vi "Result_CSVSave.vi"(11 "YTESTER测试数据":T1 caption="不要修改！") -> (3 "YTESTER结论":T2)   [LabVIEW 2017]
doc: "VIDescription=CSV格式的本地保存。"
uses:
  YtCommon.lvlibp/yt`Step StepBaseInput.ctl
  YtCommon.lvlibp/yt`Step StepResult.ctl
  YtCommon.lvlibp/yt`Step TestData.ctl
  YtCommon.lvlibp/yt`Step System Queue.ctl
  ccbe6eb8-0466-4861-8968-f05c08307fff.vi
  ac0dbf41-8066-48af-8511-23b2e407a70c.vi
  b6c5d7ee-a3f7-45be-aa43-2dbab6f386c4.vi
  YtCommon.lvlibp/yt`varSystemlib IO Read Variable.vi
  YtCommon.lvlibp
  kernel32.dll
  Advapi32.dll
panel:
  out "TiTles Array":string[](array[string])
  out "DATA array":string[](array[string])
  in  "debug":bool
  out "debug TestTable":string[][](table)
  in  "YTESTER开放参数":cluster{"YTESTER_BaseInput":T3, "保存路径":path}={"YTESTER_BaseInput"={"isTest"=FALSE, "isSkip"=FALSE, "StepName"="CSV式保存", "OnPass"=enum."Next", "OnFail"=enum."Next", "ReTestNumber"=0.0}, "保存路径"=path ""}
  # "CSV格式保存（本地）"
  # "改重入VI了！每个Socket写不同文件！"
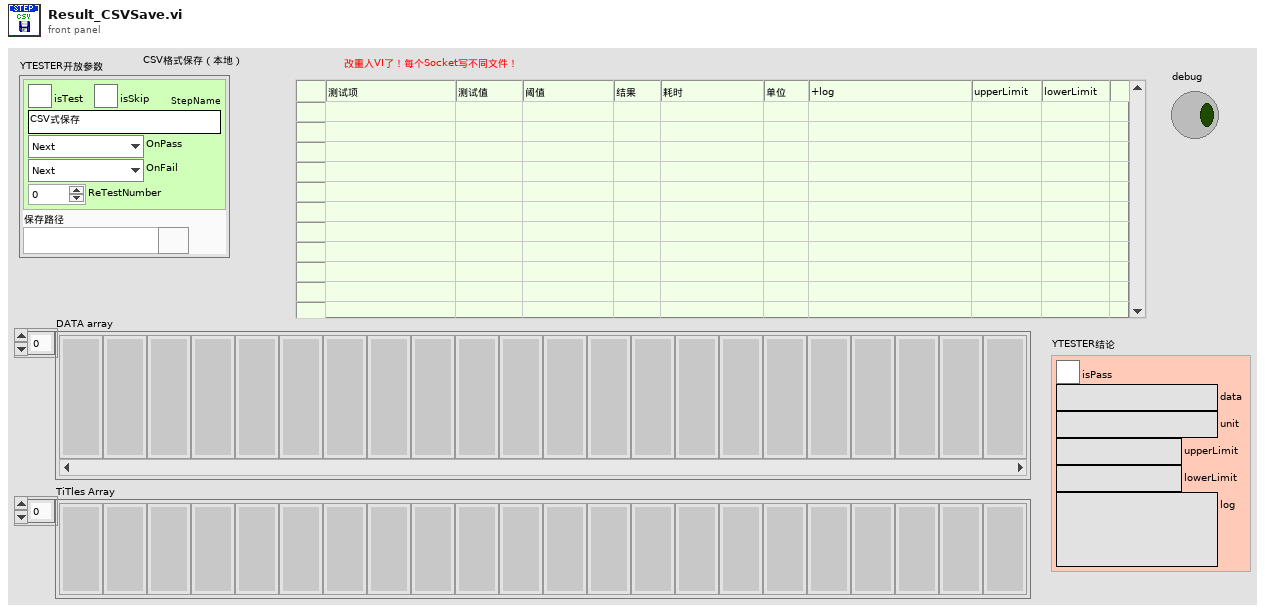
[diagram p1: front panel]
types:
  T1 = typedef "YtCommon.lvlibp/yt`Step TestData.ctl" = cluster{"Socket(From1)":i32, "SN":refnum<notifier>, "StopFlagRef":refnum<notifier>, "YT System Queue":refnum<queue>}
  T2 = typedef "YtCommon.lvlibp/yt`Step StepResult.ctl" = cluster{"isPass":bool, "data":string, "unit":string, "upperLimit":string, "lowerLimit":string, "log":string}
  T3 = typedef "YtCommon.lvlibp/yt`Step StepBaseInput.ctl" = cluster{"isTest":bool, "isSkip":bool, "StepName":string, "OnPass":enum16{"Next", "ToOVER", "Terminate"}, "OnFail":enum16{"Next", "ToOVER", "Terminate"}, "ReTestNumber":dbl}
  T4 = enum16{"open", "replace", "create", "open or create", "replace or create", "replace or create with confirmation"}
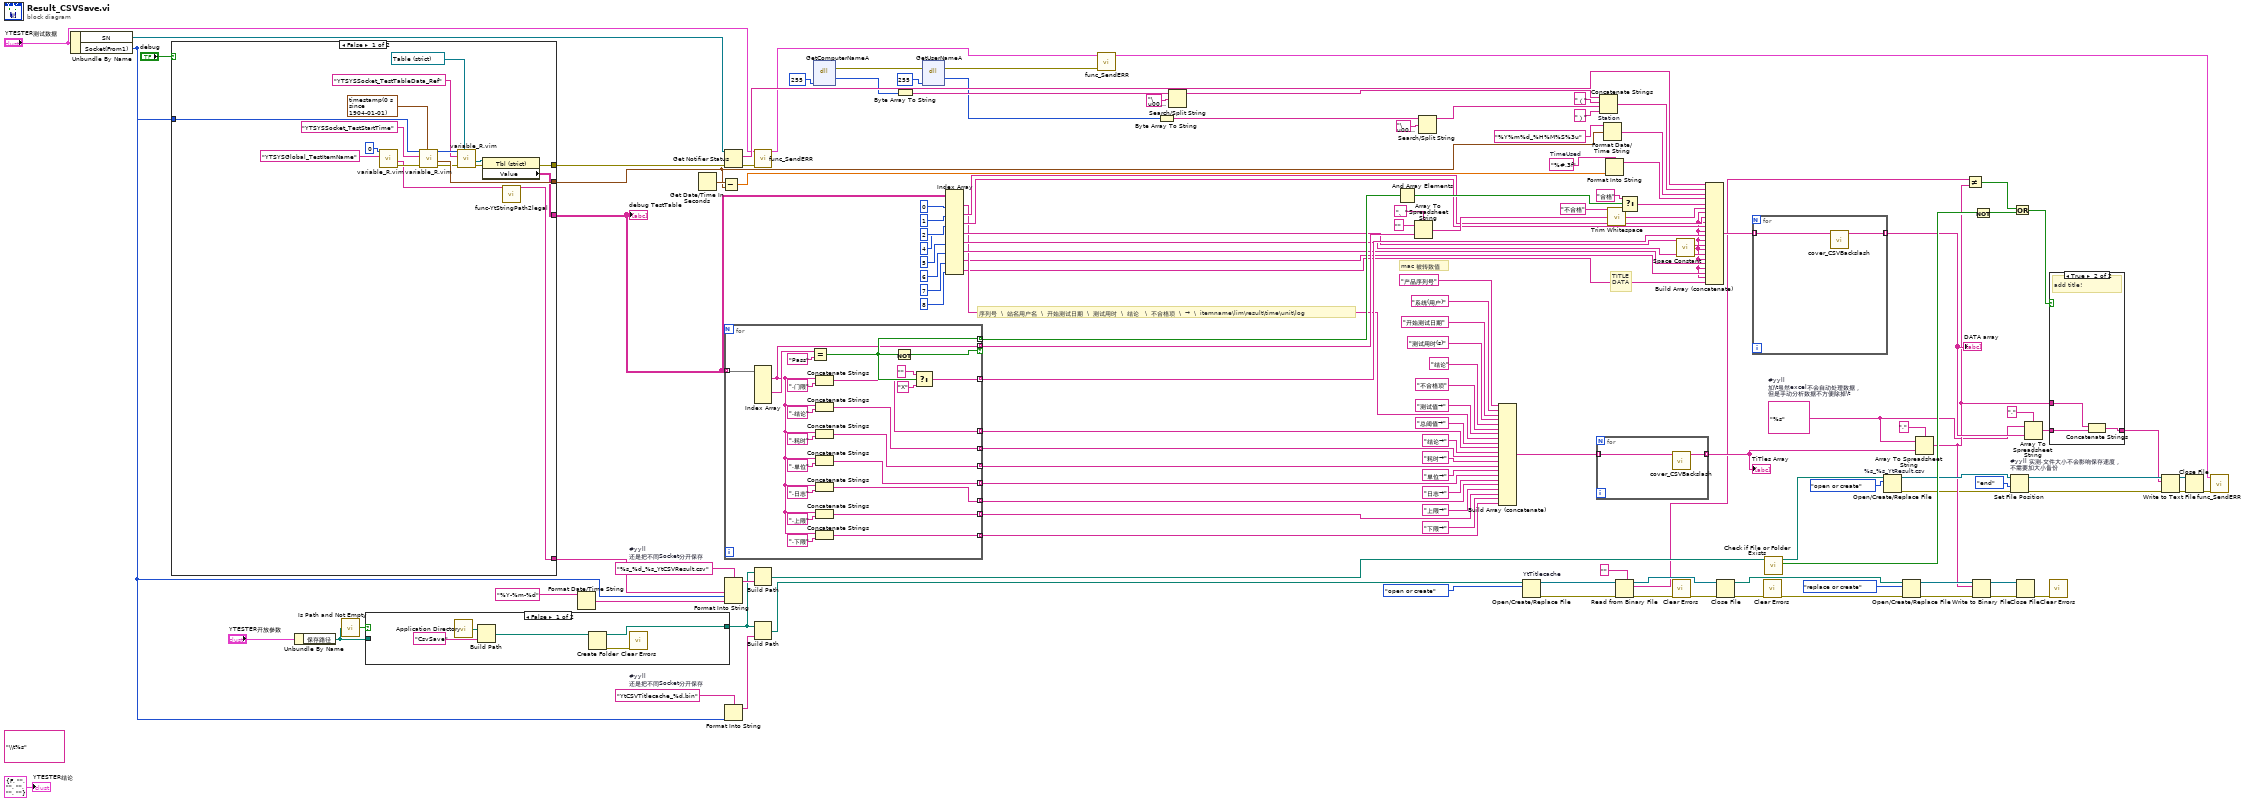
[diagram p0: block diagram]
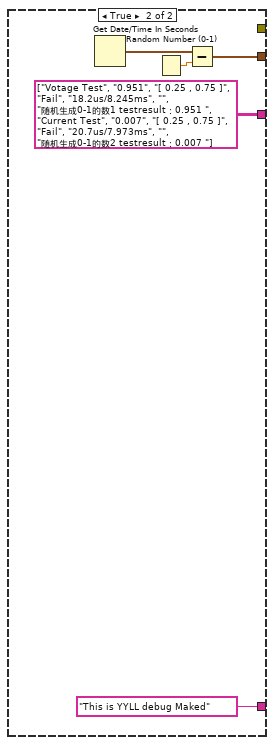
[diagram p2: hidden frame]
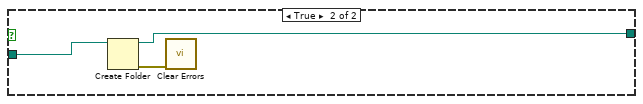
[diagram p4: hidden frame]
diagram:
  (unwired) "\\t%s" ("format string")
  w3 = "YtCSVTitlecache_%d.bin"  # #yyll 还是把不同Socket分开保存
  w15 = "%s"  # #yyll  加\t虽然excel不会自动处理数据， 但是手动分析数据不方便除掉\t
  w74 = "%s_%d_%s_YtCSVResult.csv"  # #yyll 还是把不同Socket分开保存
  w103 = "%#.3f"  # TimeUsed
  # "mac 被转数值"
  # "序列号  \\  站名用户名  \\  开始测试日期  \\  测试用时  \\  结论   \\  不合格项  \\  →  \\  itemname\\lim\\result\\time\\unit\\log"
  # "TITLE\nDATA"
  n1 = Unbundle By Name("YTESTER测试数据") -> ("SN"=w22:refnum<notifier>, "Socket(From1)"=w1:i32)
  n2 = case shown="False" "debug" {
    tunnel: [w153 "This is YYLL debug Maked"] -> w72
    tunnel: w1 -> [w152 _]
    tunnel: [w149 w156] -> w26
    tunnel: [w143 string[][] [["Votage Test", "0.951", "[ 0.25 , 0.75 ]", "Fail", "18.2us/8.245ms", "", "随机生成0-1的数1 testresult：0.951 "], ["Current Test", "0.007", "[ 0.25 , 0.75 ]", "Fail", "20.7us/7.973ms", "", "随机生成0-1的数2 testresult：0.007 "]] ("debug TestTable 2")] -> w25
    tunnel: [w137 _] -> w23
    frame False {
      n3 = call "variable_R.vim"("待获取变量名称"="YTSYSGlobal_TestItemName", "函数池名称"=0) -> ("error out"=w140:errorcluster, "value"=w138:string)  [unwired: 5 in, 3 out]
      n4 = call "variable_R.vim"("type"=timestamp(0 s since 1904-01-01), "error in"=w140, "待获取变量名称"="YTSYSSocket_TestStartTime", "函数池名称"=w152) -> ("error out"=w139:errorcluster, "value"=w149:timestamp, "函数池名称out"=w148:i32)  [unwired: 3 in, 2 out]
      n5 = call "variable_R.vim"("type"=refnum<vi> refnum ("TestTable"), "error in"=w139, "待获取变量名称"="YTSYSSocket_TestTableData_Ref", "函数池名称"=w148) -> ("error out"=w144:errorcluster, "value"=w145:refnum<vi>)  [unwired: 3 in, 3 out]
      n6 = property class="Tbl (strict)"(reference=w145, error in=w144) -> (error out=w137:errorcluster, "Value"=w143:string[][])  [unwired: 1 out]
      n7 = call "func-YtStringPath2legal.vi"("StringPath in"=w138) -> ("StringPath out"=w153:string)  [unwired: 10 in]
    }
    frame True {
      n8 = Get Date/Time In Seconds() -> (seconds since 1Jan1904=w158:timestamp)
      n9 = Random Number (0-1)() -> (number: 0 to 1=w157:dbl)
      n10 = Subtract(x=w158, y=w157) -> (x-y=w156:timestamp)
    }
  }
  "debug TestTable" <- w25
  n11 = Unbundle By Name("YTESTER开放参数") -> ("保存路径"=w133:path)
  n12 = call <vilib>:"Is Path and Not Empty.vi"("path"=w133) -> ("Is Path and Not Empty?"=w134:bool)  [unwired: 4 in]
  n13 = case shown="False" w134 {
    tunnel: w133 -> [_ w166]
    tunnel: [w160 w164] -> w38
    frame False {
      n14 = call <vilib>:"Application Directory.vi"() -> ("Application Directory"=w161:path)
      n15 = Build Path(base path=w161, name or relative path="CsvSave") -> (appended path=w163:path)
      n16 = Create Folder(path (use dialog)=w163) -> (created path=w160:path, error out=w159:errorcluster)  [unwired: 2 in, 1 out]
      n17 = call <vilib>:"Clear Errors.vi"("error in (no error)"=w159) -> ()  [unwired: 5 in, 2 out]
    }
    frame True {
      n18 = Create Folder(path (use dialog)=w166) -> (created path=w164:path, error out=w165:errorcluster)  [unwired: 2 in, 1 out]
      n19 = call <vilib>:"Clear Errors.vi"("error in (no error)"=w165) -> ()  [unwired: 5 in, 2 out]
    }
  }
  n20 = Format Date/Time String(time format string (%c)="%Y-%m-%d") -> (date/time string=w4:string)  [unwired: 1 in, 1 out]
  n21 = Get Date/Time In Seconds() -> (seconds since 1Jan1904=w105:timestamp)
  n22 = Subtract(x=w105, y=w26) -> (x-y=w104:dbl)
  n23 = Get Notifier Status(notifier=w22, error in (no error)=w23) -> (current notification=w127:string, error out=w128:errorcluster)  [unwired: 3 out]
  n24 = for {
    tunnel: w25 -> [w189] mode=indexing
    tunnel: [w185] -> w129 mode=indexing
    tunnel: [w169] -> w125 mode=indexing if=w186
    tunnel: [w182] -> w96 mode=indexing
    tunnel: [w176] -> w79 mode=indexing
    tunnel: [w175] -> w78 mode=indexing
    tunnel: [w174] -> w77 mode=indexing
    tunnel: [w173] -> w76 mode=indexing
    tunnel: [w172] -> w75 mode=indexing
    tunnel: [w168] -> w21 mode=indexing
    tunnel: [w167] -> w20 mode=indexing
    n25 = Index Array(array=w189) -> (element #1=w169:string, element #4=w188:string)  [unwired: 6 in, 4 out]
    n26 = Equal?(x=w188, y="Pass") -> (x = y?=w185:bool)
    n27 = Concatenate Strings(w169, ".门限" ("string")) -> (w176:string)
    n28 = Concatenate Strings(w169, ".结论" ("string")) -> (w175:string)
    n29 = Concatenate Strings(w169, ".耗时" ("string")) -> (w174:string)
    n30 = Concatenate Strings(w169, ".单位" ("string")) -> (w173:string)
    n31 = Concatenate Strings(w169, ".日志" ("string")) -> (w172:string)
    n32 = Concatenate Strings(w169, ".上限" ("string")) -> (w168:string)
    n33 = Concatenate Strings(w169, ".下限" ("string")) -> (w167:string)
    n34 = Not(x=w185) -> (.not. x?=w186:bool)
    n35 = Select(t="" ("y"), s=w185, f="Ⅹ" ("y")) -> (s? t:f=w182:string)
  }
  n36 = Format Into String(format string=w74, w72, w1, w4) -> (resulting string=w71:string)  [unwired: 2 in, 1 out]
  n37 = Format Into String(format string=w3, w1) -> (resulting string=w2:string)  [unwired: 2 in, 1 out]
  n38 = call "func_SendERR.vi"("ERR (String\\Errclust)"=w128, "YTESTER测试数据 in"="YTESTER测试数据") -> ("YTESTER测试数据 out"=w31:T1)  [unwired: 9 in]
  n39 = Build Path(base path=w38, name or relative path=w71) -> (appended path=w60:path)
  n40 = Build Path(base path=w38, name or relative path=w2) -> (appended path=w39:path)
  n41 = dll-call lib="kernel32.dll" fn="GetComputerNameA" label="Get Computer Name"("size"=255) -> (error out=w33:errorcluster, "lpBuffer"=w120:u8[])  [unwired: 6 in, 1 out]
  n42 = Byte Array To String(unsigned byte array=w120) -> (string=w119:string)
  n43 = dll-call lib="advapi32.dll" fn="GetUserNameA" label="GetUserName"(error in=w33, "nSize"=u32 255) -> (error out=w32:errorcluster, "lpBuffer"=w116:u8[])  [unwired: 5 in, 1 out]
  n44 = Index Array(array=w25, index (col) #1=0 ("disabled index (col)"), index (col) #2=1 ("index (col)"), index (col) #3=2 ("index (col)"), index (col) #4=4 ("index (col)"), index (col) #5=5 ("index (col)"), index (col) #6=6 ("index (col)"), index (col) #7=7 ("index (col)"), index (col) #8=8 ("index (col)")) -> (element #1=w80:string[], element #2=w99:string[], element #3=w97:string[], element #4=w94:string[], element #5=w91:string[], element #6=w90:string[], element #7=w17:string[], element #8=w16:string[])  [unwired: 8 in]
  n45 = call "func_SendERR.vi"("ERR (String\\Errclust)"=w32, "YTESTER测试数据 in"=w31) -> ("YTESTER测试数据 out"=w30:T1)  [unwired: 9 in]
  n46 = Byte Array To String(unsigned byte array=w116) -> (string=w115:string)
  n47 = Search/Split String(string=w119, search string/char (-)="\u0000" ("regular expression")) -> (substring before match=w112:string)  [unwired: 1 in, 2 out]
  n48 = And Array Elements(Boolean array=w129) -> (logical AND=w132:bool)
  n49 = Array To Spreadsheet String(delimiter (Tab)="、", array=w125, 3:"" ("format string")) -> (spreadsheet string=w122:string)
  n50 = Search/Split String(string=w115, search string/char (-)="\u0000" ("regular expression")) -> (substring before match=w110:string)  [unwired: 1 in, 2 out]
  n51 = Build Array (concatenate) ("Build DATA Array")("产品序列号", "系统(用户)", "开始测试日期", "测试用时(s)", "结论", "不合格项", "测试值→", w80, "总阈值→", w79, "结论→", w78, "耗时→", w77, "单位→", w76, "日志→", w75, "上限→", w21, "下限→", w20) -> (w87:string[])
  n52 = Open/Create/Replace File "YtTitlecache"(file path (use dialog)=w39, operation (0:open)=T4."open or create") -> (refnum out=w51:refnum<file>, error out=w54:errorcluster)  [unwired: 4 in, 1 out]
  n53 = for {
    tunnel: [w191] -> w55 mode=indexing
    tunnel: w87 -> [w190] mode=indexing
    n54 = call "cover_CSVBackslash.vi"("String in"=w190) -> ("String out"=w191:string)  [unwired: 10 in]
  }
  "TiTles Array" <- w55
  n55 = Concatenate Strings "Station"(w112, "（" ("string"), w110, "）" ("string")) -> (w108:string)
  n56 = Format Date/Time String(time format string (%c)="%Y%m%d_%H%M%S%3u", seconds (now)=w26) -> (date/time string=w106:string)  [unwired: 1 in]
  n57 = Format Into String(format string=w103, w104) -> (resulting string=w102:string)  [unwired: 2 in, 1 out]
  n58 = call <vilib>:"Trim Whitespace.vi"("string"=w122) -> ("trimmed string"=w121:string)  [unwired: 1 in]
  n59 = Read from Binary File(5:"", 8:w54, 11:w51) -> (0:w48:errorcluster, 2:w36:string, 3:w49:refnum<file>)  [unwired: 3 in, 1 out]
  n60 = Select(t="合格", s=w132, f="不合格") -> (s? t:f=w126:string)
  n61 = call <vilib>:"Clear Errors.vi"("error in (no error)"=w48) -> ("error out"=w43:errorcluster)  [unwired: 5 in, 1 out]
  n62 = call <vilib>:"Space Constant.vi"() -> ("String"=w7:string)
  n63 = Build Array (concatenate) ("Build DATA Array")(w127, w108, w106, w102, w126, w121, w7, w99, w7, w97, w7, w96, w7, w94, w7, w91, w7, w90, w7, w17, w7, w16) -> (w89:string[])
  n64 = Close File(refnum=w49, error in=w43) -> (path=w46:path, error out=w41:errorcluster)
  n65 = for {
    tunnel: w89 -> [w193] mode=indexing
    tunnel: [w192] -> w58 mode=indexing
    n66 = call "cover_CSVBackslash.vi"("String in"=w193) -> ("String out"=w192:string)  [unwired: 10 in]
  }
  "DATA array" <- w58
  n67 = call <vilib>:"Clear Errors.vi"("error in (no error)"=w41) -> ("error out"=w40:errorcluster)  [unwired: 5 in, 1 out]
  n68 = call <vilib>:"Check if File or Folder Exists.vi"("path"=w60) -> ("file or folder exists?"=w67:bool, "dup path"=w66:path)  [unwired: 8 in, 1 out]
  n69 = Open/Create/Replace File "%s_%s_YtResult.csv"(file path (use dialog)=w66, operation (0:open)=T4."open or create") -> (refnum out=w65:refnum<file>, error out=w29:errorcluster)  [unwired: 4 in, 1 out]
  n70 = Open/Create/Replace File(file path (use dialog)=w46, error in=w40, operation (0:open)=T4."replace or create") -> (refnum out=w45:refnum<file>, error out=w47:errorcluster)  [unwired: 3 in, 1 out]
  n71 = Array To Spreadsheet String(delimiter (Tab)=",", array=w55, 3:w15) -> (spreadsheet string=w34:string)
  n72 = Not Equal?(x=w36, y=w34) -> (x != y?=w35:bool)
  n73 = Write to Binary File(file (use dialog)=w45, data=w34, error in=w47) -> (refnum out=w53:refnum<file>, error out=w52:errorcluster)  [unwired: 3 in, 1 out]
  n74 = Not(x=w67) -> (.not. x?=w62:bool)
  n75 = Set File Position "#yyll 实测,文件大小不会影响保存速度，\n不需要加大小备份"(refnum=w65, from (0:start)=enum16{"start", "end", "current"}."end", error in=w29) -> (refnum out=w68:refnum<file>, error out=w69:errorcluster)  [unwired: 1 in]
  n76 = Or(x=w35, y=w62) -> (x .or. y?=w61:bool)
  n77 = Close File(refnum=w53, error in=w52) -> (error out=w42:errorcluster)  [unwired: 1 out]
  n78 = Array To Spreadsheet String(delimiter (Tab)=",", array=w58, 3:w15) -> (spreadsheet string=w57:string)
  n79 = case shown="True" w61 {
    tunnel: w57 -> [w194 w197]
    tunnel: [w194 w196] -> w63
    tunnel: w34 -> [_ w195]
    frame False {
    }
    frame True {
      # "add title!"
      n80 = Concatenate Strings(w195, w197) -> (w196:string)
    }
  }
  n81 = call <vilib>:"Clear Errors.vi"("error in (no error)"=w42) -> ()  [unwired: 5 in, 2 out]
  n82 = Write to Text File(file (use dialog)=w68, text=w63, error in=w69) -> (refnum out=w6:refnum<file>, error out=w5:errorcluster)  [unwired: 1 in, 1 out]
  n83 = Close File(refnum=w6, error in=w5) -> (error out=w28:errorcluster)  [unwired: 1 out]
  n84 = call "func_SendERR.vi"("ERR (String\\Errclust)"=w28, "YTESTER测试数据 in"=w30) -> ()  [unwired: 9 in, 1 out]
  "YTESTER结论" <- T2 {"isPass"=FALSE, "data"="", "unit"="", "upperLimit"="", "lowerLimit"="", "log"=""} ("Result")
